vi "list dir.vi"(8 "error in (no error)":errorcluster, 10 "path":string, 11 "TCP in":refnum<k5>) -> (0 "error out":errorcluster, 2 "Array":T1[](array[typedef]), 3 "TCP out":refnum<k5>)   [LabVIEW 2020]
uses:
  ctl/0-id,name.ctl
  ctl/9-id,name,path.ctl
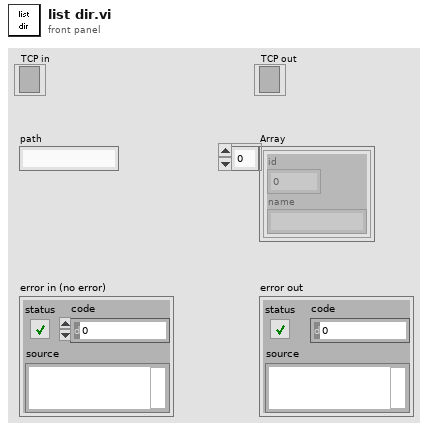
[diagram p1: front panel]
types:
  T1 = typedef "0-id,name.ctl" = cluster{"id":u8, "name":string}
  T2 = typedef "9-id,name,path.ctl" = cluster{"id":u8, "name":string, "path":string}
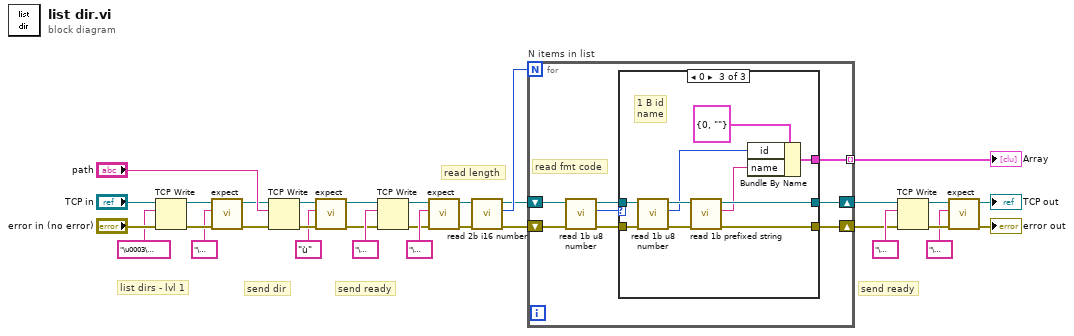
[diagram p0: block diagram]
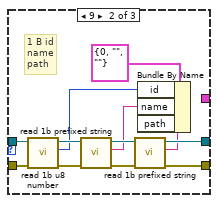
[diagram p3: hidden frame]
diagram:
  # "send ready"
  # "send ready"
  # "send dir"
  # "read length"
  # "list dirs - lvl 1"
  n1 = TCP Write(connection ID="TCP in", data in="\u0003\u0000\u0001", error in (no error)="error in (no error)") -> (connection ID out=w15:refnum<k5>, error out=w17:errorcluster)  [unwired: 1 in, 1 out]
  n2 = call "expect.vi"("error in (no error)"=w17, "data expected"="\u0001" ("data in"), "TCP Network Connection in"=w15) -> ("error out"=w16:errorcluster, "TCP Network Connection out"=w21:refnum<k5>)  [unwired: 6 in, 1 out]
  n3 = TCP Write(connection ID=w21, data in="path", error in (no error)=w16) -> (connection ID out=w26:refnum<k5>, error out=w25:errorcluster)  [unwired: 1 in, 1 out]
  n4 = call "expect.vi"("error in (no error)"=w25, "data expected"="ù" ("data in"), "TCP Network Connection in"=w26) -> ("error out"=w24:errorcluster, "TCP Network Connection out"=w27:refnum<k5>)  [unwired: 6 in, 1 out]
  n5 = TCP Write(connection ID=w27, data in="\u0001", error in (no error)=w24) -> (connection ID out=w31:refnum<k5>, error out=w29:errorcluster)  [unwired: 1 in, 1 out]
  n6 = call "expect.vi"("error in (no error)"=w29, "data expected"="\u0001" ("data in"), "TCP Network Connection in"=w31) -> ("error out"=w4:errorcluster, "TCP Network Connection out"=w5:refnum<k5>)  [unwired: 6 in, 1 out]
  n7 = call "read 2b i16 number.vi"("error in (no error)"=w4, "TCP Network Connection in"=w5) -> ("error out"=w1:errorcluster, "number"=w3:i16, "TCP Network Connection out"=w2:refnum<k5>)  [unwired: 7 in]
  n8 = for "N items in list" {
    N: w3 -> [_]
    shift-right: [w35] -> w8
    shift-left: w2 -> [w40]
    shift-right: [w37] -> w9
    shift-left: w1 -> [w39]
    tunnel: [w33] -> w32 mode=indexing
    # "read fmt code"
    n9 = call "read 1b u8 number.vi"("error in (no error)"=w39, "TCP Network Connection in"=w40) -> ("error out"=w38:errorcluster, "number"=w34:u8, "TCP Network Connection out"=w36:refnum<k5>)  [unwired: 7 in]
    n10 = case shown="0" w34 {
      tunnel: w38 -> [w41 w54 w64]
      tunnel: [w41 w48 w59] -> w37
      tunnel: w36 -> [w42 w50 w61]
      tunnel: [w42 w46 w58] -> w35
      tunnel: [_ _ w55] -> w33
      frame Default {
      }
      frame 9 {
        # "1 B id\nname\npath"
        n11 = call "read 1b u8 number.vi"("error in (no error)"=w54, "TCP Network Connection in"=w50) -> ("error out"=w51:errorcluster, "number"=w45:u8, "TCP Network Connection out"=w49:refnum<k5>)  [unwired: 7 in]
        n12 = call "read 1b prefixed string.vi"("error in (no error)"=w51, "TCP Network Connection in"=w49) -> ("error out"=w53:errorcluster, "data out"=w44:string, "TCP Network Connection out"=w47:refnum<k5>)  [unwired: 7 in]
        n13 = call "read 1b prefixed string.vi"("error in (no error)"=w53, "TCP Network Connection in"=w47) -> ("error out"=w48:errorcluster, "data out"=w43:string, "TCP Network Connection out"=w46:refnum<k5>)  [unwired: 7 in]
        n14 = Bundle By Name(cluster=T2 {"id"=0, "name"="", "path"=""} ("9 - id, len, data"), "id"=w45, "name"=w44, "path"=w43) -> ()  [unwired: 1 out]
      }
      frame 0 {
        # "1 B id\nname"
        n15 = call "read 1b u8 number.vi"("error in (no error)"=w64, "TCP Network Connection in"=w61) -> ("error out"=w62:errorcluster, "number"=w57:u8, "TCP Network Connection out"=w60:refnum<k5>)  [unwired: 7 in]
        n16 = call "read 1b prefixed string.vi"("error in (no error)"=w62, "TCP Network Connection in"=w60) -> ("error out"=w59:errorcluster, "data out"=w56:string, "TCP Network Connection out"=w58:refnum<k5>)  [unwired: 7 in]
        n17 = Bundle By Name(cluster=T1 {"id"=0, "name"=""} ("9 - id, len, data"), "id"=w57, "name"=w56) -> (w55:T1)
      }
    }
  }
  "Array" <- w32
  n18 = TCP Write(connection ID=w8, data in="\u0001", error in (no error)=w9) -> (connection ID out=w10:refnum<k5>, error out=w12:errorcluster)  [unwired: 1 in, 1 out]
  n19 = call "expect.vi"("error in (no error)"=w12, "data expected"="\u0001" ("data in"), "TCP Network Connection in"=w10) -> ("error out"=→"error out":errorcluster, "TCP Network Connection out"=→"TCP out":refnum<k5>)  [unwired: 6 in, 1 out]
